vi "W9EO82,FBO8PP_5.vi"() -> ()   [LabVIEW 2021]
uses:
  <vilib>/measure/NI_MABase.lvlib
panel:
  out "V effektiv":dbl
  out "Integral":dbl
  out "?":string
  out "?":string
  out "?":string
  out "?":string
  in  "Slide":i32(slide) scale=0.0..3.0
  out "Waveform Graph":waveform(dbl)(graph)
  in  "offset":dbl format="%0.2p"
  in  "amplitudo":dbl=1.0 format="%0.2p"
  in  "frekvencia":dbl=10.0 format="%0.2p"
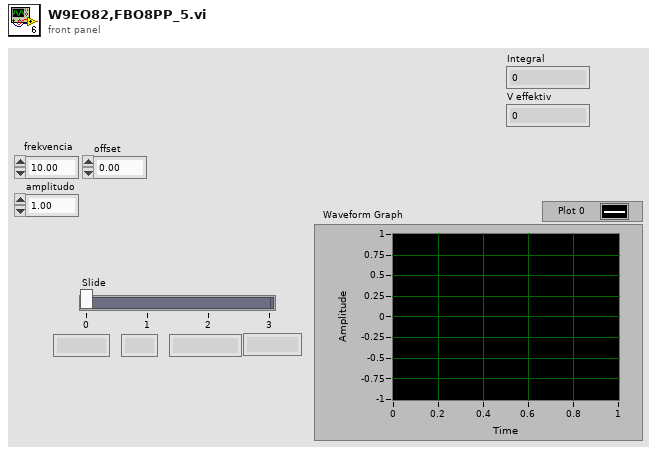
[diagram p1: front panel]
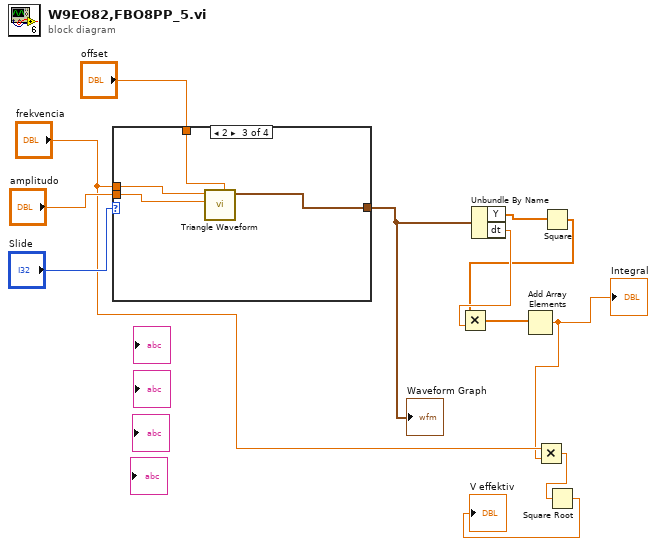
[diagram p0: block diagram]
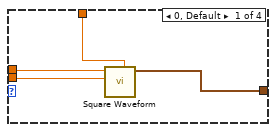
[diagram p2: hidden frame]
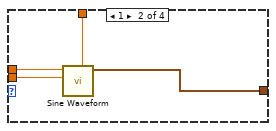
[diagram p3: hidden frame]
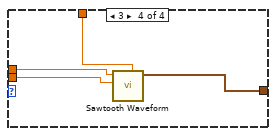
[diagram p4: hidden frame]
diagram:
  n1 = case shown="2" "Slide" {
    tunnel: "frekvencia" -> [w16 w20 w24 w28]
    tunnel: "amplitudo" -> [w15 w19 w23 w27]
    tunnel: "offset" -> [w14 w18 w22 w26]
    tunnel: [w13 w17 w21 w25] -> w9
    frame 0, Default {
      n2 = call <vilib>:"Square Waveform.vi"("offset"=w14, "amplitude"=w15, "frequency"=w16) -> ("signal out"=w13:waveform(dbl))  [unwired: 7 in, 1 out]
    }
    frame 1 {
      n3 = call <vilib>:"Sine Waveform.vi"("offset"=w18, "amplitude"=w19, "frequency"=w20) -> ("signal out"=w17:waveform(dbl))  [unwired: 7 in, 1 out]
    }
    frame 2 {
      n4 = call <vilib>:"Triangle Waveform.vi"("offset"=w22, "amplitude"=w23, "frequency"=w24) -> ("signal out"=w21:waveform(dbl))  [unwired: 7 in, 1 out]
    }
    frame 3 {
      n5 = call <vilib>:"Sawtooth Waveform.vi"("offset"=w26, "amplitude"=w27, "frequency"=w28) -> ("signal out"=w25:waveform(dbl))  [unwired: 7 in, 1 out]
    }
  }
  "Waveform Graph" <- w9
  n6 = Unbundle By Name(w9) -> ("Y"=w3:dbl[], "dt"=w8:dbl)
  n7 = Square(x=w3) -> (x^2=w2:dbl[])
  n8 = Multiply(x=w2, y=w8) -> (x*y=w1:dbl[])
  n9 = Add Array Elements(numeric array=w1) -> (sum=w4:dbl)
  "Integral" <- w4
  n10 = Multiply(x="frekvencia", y=w4) -> (x*y=w6:dbl)
  n11 = Square Root(x=w6) -> (sqrt(x)=→"V effektiv":dbl)
